vi "Trav_single_profile.vi"(3 "Simulate/Run":T1, 5 "Traverse line":T2 {"Carrier_2 Q (l/min)" format="%#.2f"; "Row Duration (mins)" format="%#.1f"; "Row No" min=0; "Trace Gas Concentration (%)" min=0.0 format="%#_4f"; "Carrier_1 Q (l/min)" format="%#.2f"; "Tunnel Speed" format="%#.2f"; "Start X" format="%#.2f"; "Start Y" format="%#.2f"; "Start Z" format="%#.2f"; "End X" format="%#.2f"; "End Y" format="%#.2f"; "End Z" format="%#.2f"; "Averaging time (min)" min=0.0 format="%#.2f"}) -> (0 "Error Messages":string, 1 "Status":T5, 2 "Traverse line Out":T2 {"Carrier_2 Q (l/min)" format="%#.2f"; "Row Duration (mins)" format="%#.1f"; "Row No" min=0; "Trace Gas Concentration (%)" min=0.0 format="%#_4f"; "Carrier_1 Q (l/min)" format="%#.2f"; "Tunnel Speed" format="%#.2f"; "Start X" format="%#.2f"; "Start Y" format="%#.2f"; "Start Z" format="%#.2f"; "End X" format="%#.2f"; "End Y" format="%#.2f"; "End Z" format="%#.2f"; "Averaging time (min)" min=0.0 format="%#.2f"})   [LabVIEW 2015]
uses:
  Gen Trav/Multi_Run_Status.ctl
  Gen Trav/Traverse_cluster.ctl
  Gen Trav/Spacing.ctl
  Controls/Multi_run_mode.ctl
  Controls/User_Specific_mode.ctl
  Controls/Overhead.ctl
  Controls/Setup.ctl
  Controls/Save_Data.ctl
  Camera Server/Camera enum/Camera resolution.ctl
  ADAM Client/Sub VIs/ADAM Controls/Traverse_Level_State.ctl
  Globals/Extra_Commands_Global.vi
  Globals/Trav_pos_global.vi
  Globals/Meas_global.vi
panel:
  out "Pause message":string
  in  "Pause":bool
  out "Current position":sgl[](array[numeric]) format="%.2f"
  in  "Stop":bool
  in  "Array of Positions":sgl[][](array[numeric]) format="%.2f"
  out "Abcissa copy":string="Y (mm)"
  out "Abcissa":string="Y (mm)"
  in  "ChannelsToPlot":i32[](listbox)=[1]
  out "Started Profile at:":string="16/9/98 12:33"
  out "Currently on point":i32=9
  out "Means":cluster{sgl[], sgl[]}[](graph)
  out "Turbulence%":cluster{sgl[], sgl[]}[](graph)
  # "X           Y            Z"
  # "Start"
  # "End"
  # "X           Y            Z"
  # "Start"
  # "End"
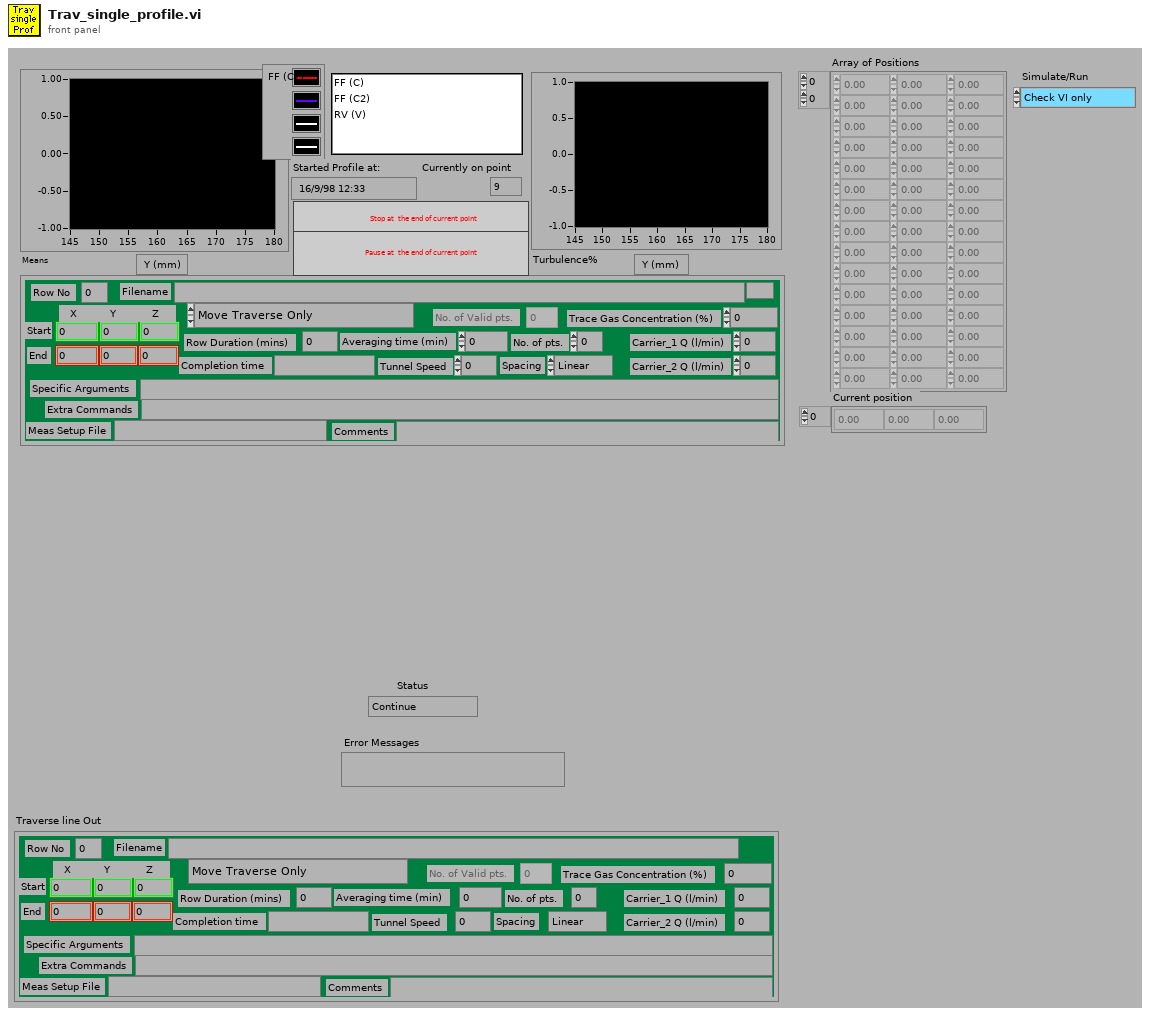
[diagram p1: front panel]
types:
  T1 = typedef "User_Specific_mode.ctl" = enum16{"Check VI only", "Run VI"}
  T2 = typedef "Traverse_cluster.ctl" = cluster{"Start X":sgl, "Start Y":sgl, "Start Z":sgl, "End X":sgl, "End Y":sgl, "End Z":sgl, "No. of pts.":i32, "Spacing":T3, "Filename":path, "Tunnel Speed":dbl, "Averaging time (min)":dbl, "Extra Commands":string, "Carrier_1 Q (l/min)":dbl, "Carrier_2 Q (l/min)":dbl, "Trace Gas Concentration (%)":dbl, "Specific Arguments":string, "Comments":string, "Row No":i32, "Row Type Selector":T4, "Completion time":string, "Row Duration (mins)":dbl, "No. of Valid pts.":i32, "Meas Setup File":string}
  T3 = typedef "Spacing.ctl" = enum16{"Linear", "Log", "Gauss", "Specified", "N/A"}
  T4 = typedef "Multi_run_mode.ctl" = enum16{"Move Traverse Only", "Set Tunnel Speed Only", "Set Source Only", "Set Measurement Conditions", "Single Measurement", "Vertical Profile", "Lateral Profile", "Longitudinal Profile", "Explore Volume", "Multi-Axis Profile", "Auto Calibrate", "Meas Fast FID Bkgnd", "Check Beam Power", "Scanning Valve Measurement", "Run VI Named:", "Set ADAM Ch", "Wait (minutes)", "Send Message", "Synchronize With:", "Fall Back to this Row", "Turn Off Row Repeating", "Blank Row", "Traverse 3D Volume"}
  T5 = typedef "Multi_Run_Status.ctl" = enum16{"Continue", "Jump to Next Point", "Jump to Next Row", "Jump To Fall Back", "Terminate Run"}
  T6 = typedef "Overhead.ctl" = enum16{"Update total times", "Read Current Overhead", "Re Scale totals to 3 hrs", "Initialise totals to 3hr"}
  T7 = typedef "Save_Data.ctl" = enum16{"Save No Data", "Save Data"}
  T8 = typedef "Setup.ctl" = enum16{"Run Program", "Show Setup", "Save Current Setup", "Setup Front Panel"}
  T9 = typedef "Traverse_Level_State.ctl" = enum16{"Running", "Complete"}
  T10 = typedef "Status_Cluster.ctl" = cluster{"Status":T5, "Error Type":string, "Error Description":string}
  T11 = typedef "Camera resolution.ctl" = u8
  T12 = typedef "Analysis_info_cluster.ctl" = cluster{"Colour":u32, "Inst type":T13, "Inst name":string, "Symbol":string, "Code name":string, "Extra Info":string, "Inst Array":T14, "Extra Titles":string[], "Extra Values":string[], "U":dbl, "u^2":dbl, "u^3":dbl, "u^4":dbl, "Skew_u":dbl, "Kurt_u":dbl, "Sd Error in Mean":dbl, "% u'/U":dbl, "X":dbl, "Y":dbl, "Z":dbl, "Timescale integral to 25%":dbl, "Sd Error in Variance":dbl, "Calib File":path, "Calib Constants":dbl[], "Output Position":bool, "Full Stats":bool, "Av Sampling Rate":dbl, "Av No of Samples":dbl, "Total Meas Time (s)":dbl, "ADAM Ch Name":string, "Max value":dbl, "Min value":dbl}
  T13 = typedef "Inst_type.ctl" = enum16{"Propeller anemometer", "Raw voltage", "Pressure Transducer", "Pitot-static tube", "Preston tube", "Hot wire", "Cross wire 1", "Cross wire 2", "Generic Linear", "Generic Polynomial", "Generic BackPoly", "Fast FID", "Thermocouple", "Cold wire", "Pulsed Wire", "LDA Vel", "LDA Tran time", "LDA Arr time", "Microphone"}
  T14 = typedef "Instrument_Array.ctl" = enum16{"PWA", "LDA", "Analogue"}
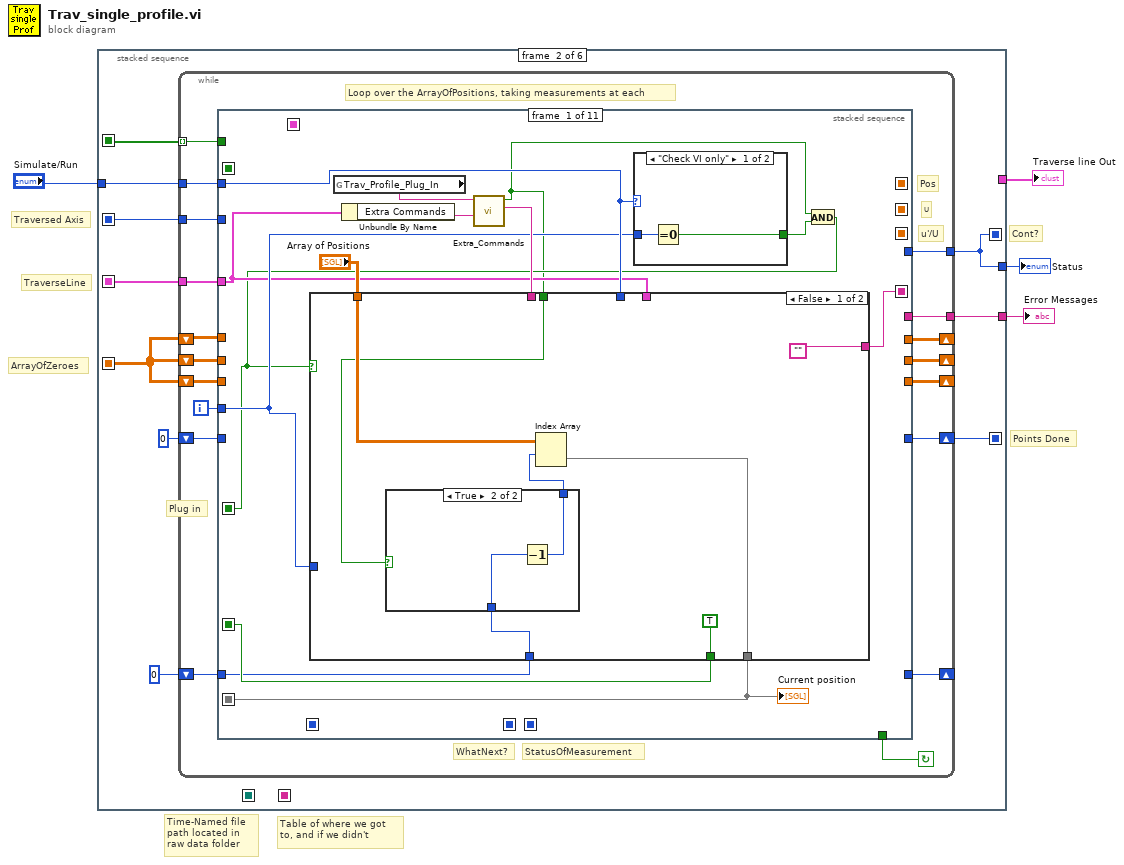
[diagram p0: block diagram]
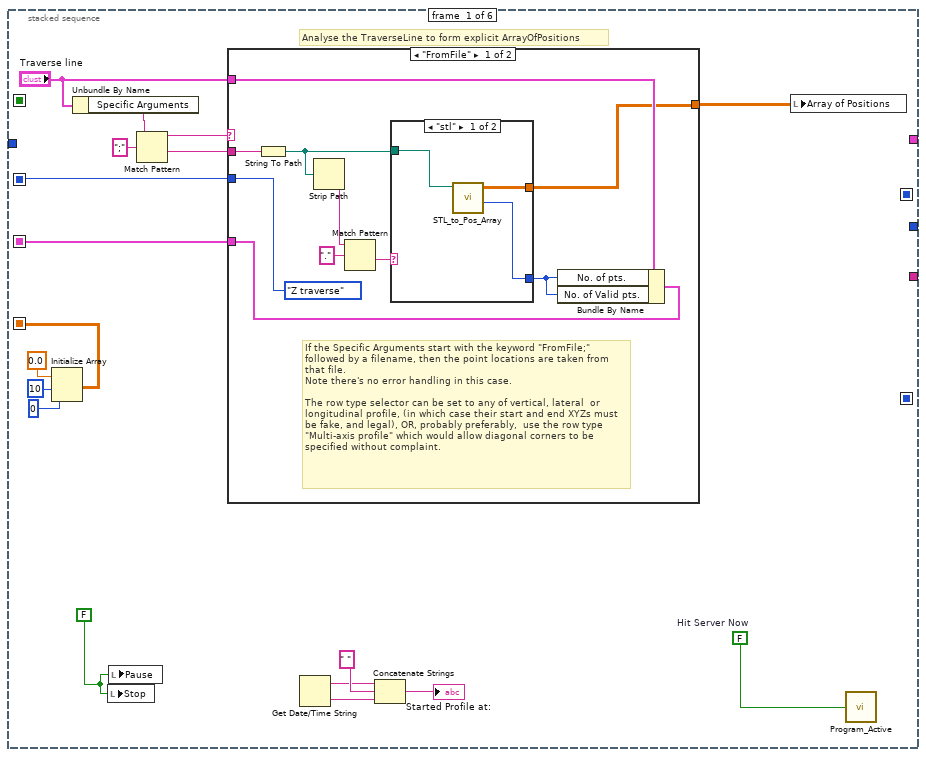
[diagram p2: hidden frame]
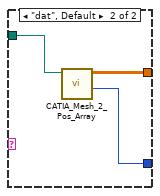
[diagram p3: hidden frame]
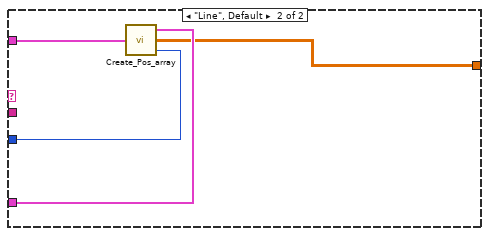
[diagram p4: hidden frame]
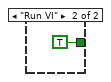
[diagram p5: hidden frame]
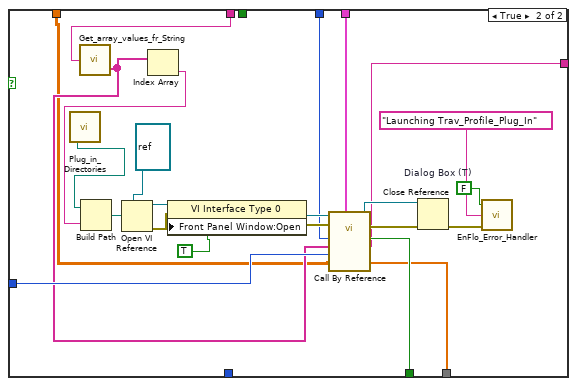
[diagram p7: hidden frame]
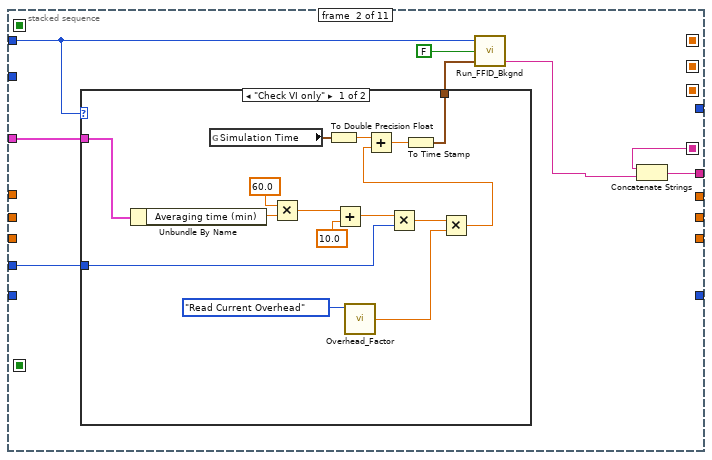
[diagram p8: hidden frame]
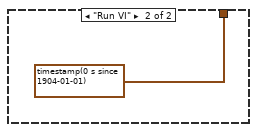
[diagram p9: hidden frame]
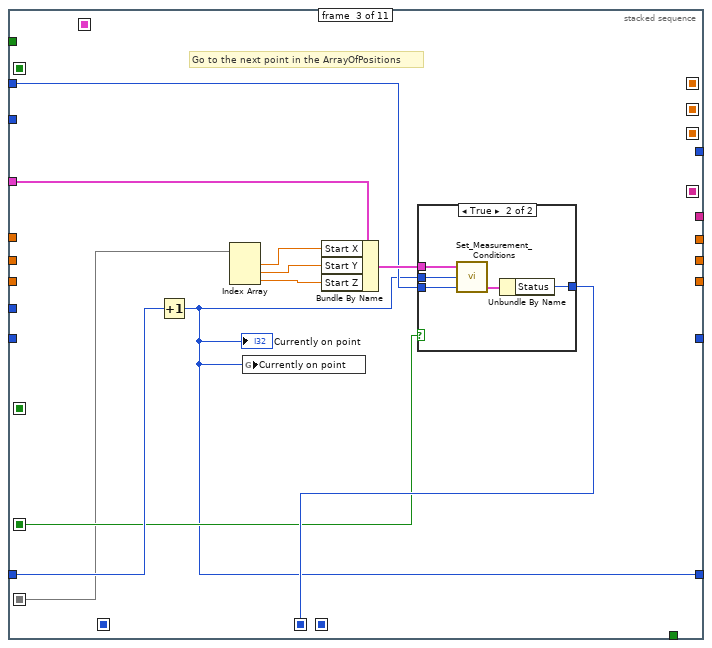
[diagram p10: hidden frame]
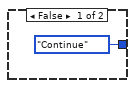
[diagram p11: hidden frame]
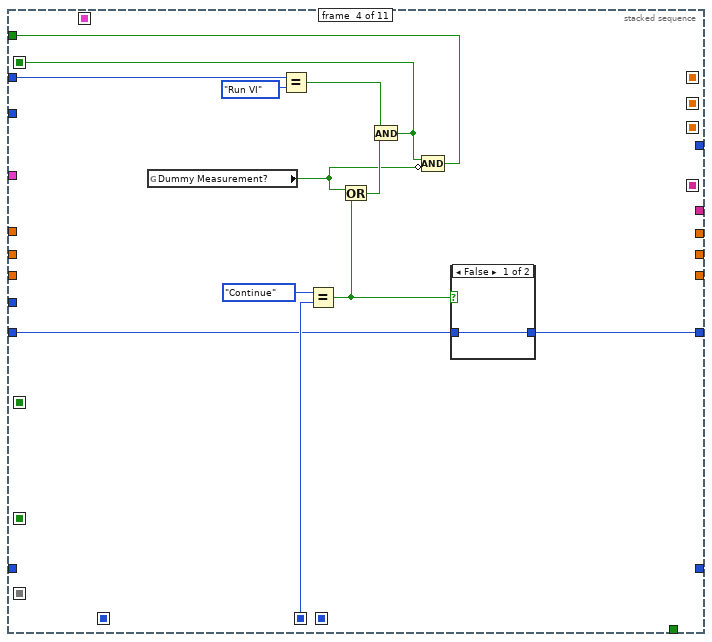
[diagram p12: hidden frame]
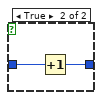
[diagram p13: hidden frame]
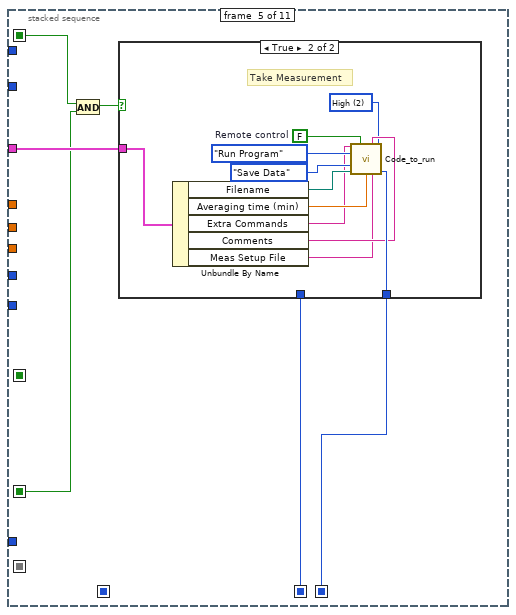
[diagram p14: hidden frame]
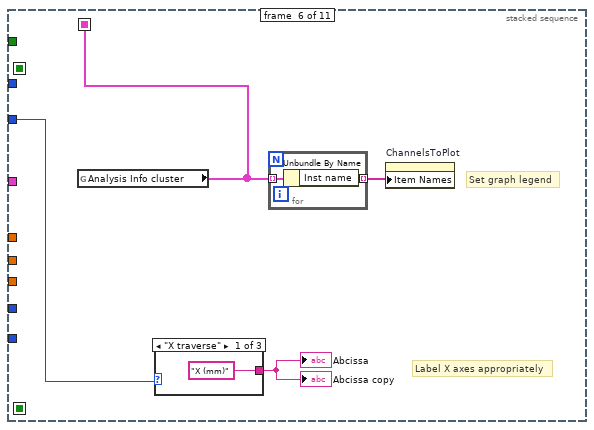
[diagram p16: hidden frame]
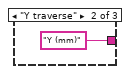
[diagram p17: hidden frame]
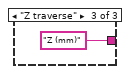
[diagram p18: hidden frame]
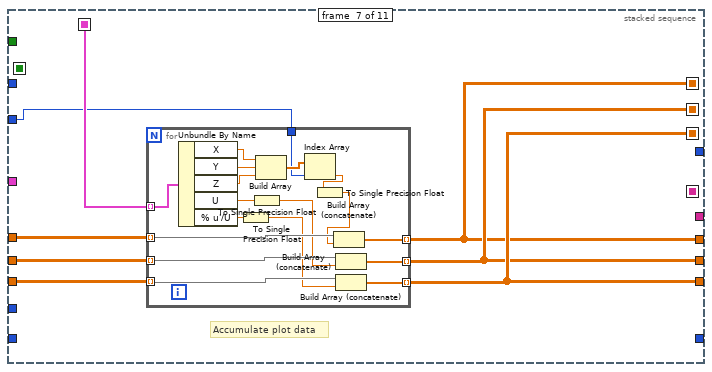
[diagram p19: hidden frame]
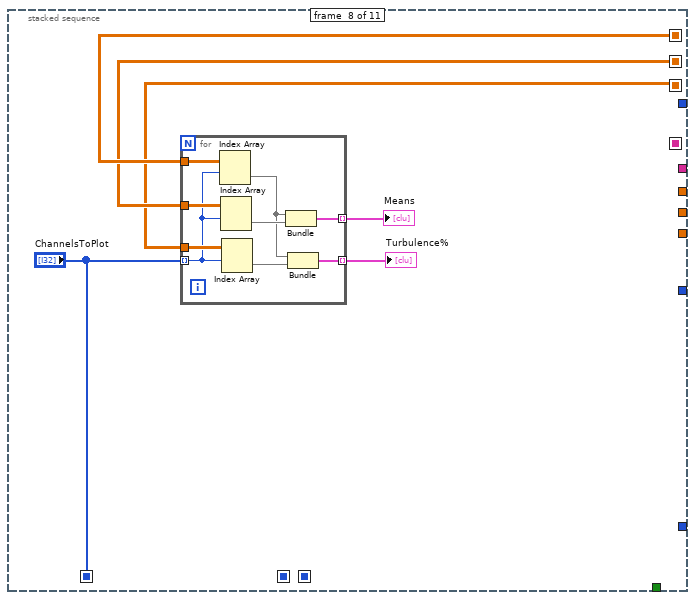
[diagram p20: hidden frame]
diagram:
  # "Table of where we got to, and if we didn't"
  # "Time-Named file path located in raw data folder"
  # "ArrayOfZeroes"
  # "TraverseLine"
  # "Traversed Axis"
  # "Points Done"
  # "Cont?"
  n1 = stacked-sequence {
    seq-local: [w15 _ _ _ _ _] -> [_ w51 _ _ _ _]
    seq-local: [w14 _ _ _ _ _] -> [_ w52 _ _ _ _]
    seq-local: [_ _ w335 _ _ _] -> [_ _ _ _ w359 _]
    seq-local: [_ _ _ w342 _ _] -> [_ _ _ _ w358 _]
    seq-local: [_ w50 _ _ _ _] -> [_ _ _ _ _ _]
    seq-local: [_ w48 _ _ _ _] -> [_ _ _ w339 w357 _]
    seq-local: [_ w46 _ _ _ _] -> [_ _ _ _ _ w364]
    seq-local: [w11 _ _ _ _ _] -> [_ w45 _ _ _ w366]
    tunnel: [_ w50 _ _ _ _] -> w2
    tunnel: [_ _ _ _ _ w376] -> w4
    tunnel: "Simulate/Run" -> [_ w49 _ _ _ w375]
    tunnel: [_ w44 _ _ _ _] -> w1
    frame #0 {
      w12 = FALSE ("stop")
      w13 = FALSE  # Hit Server Now
      # "Analyse the TraverseLine to form explicit ArrayOfPositions"
      n2 = Initialize Array(sgl 0.0, 10, 0) -> (w15:sgl[][])
      n3 = Unbundle By Name("Traverse line") -> ("Specific Arguments"=w8:string)
      n4 = local write "Stop"(w12) -> ()
      n5 = local write "Pause"(w12) -> ()
      n6 = Match Pattern(string=w8, regular expression=";") -> (before substring=w6:string, after substring=w5:string)  [unwired: 1 in, 2 out]
      n7 = case shown="\"FromFile\"" w6 {
        tunnel: [enum16{"X traverse", "Y traverse", "Z traverse"}."Z traverse" ("Axis Traversed") w42] -> w14
        tunnel: "Traverse line" -> [w26 w41]
        tunnel: [w25 w40] -> w11
        tunnel: [w23 w39] -> w10
        tunnel: w5 -> [w27 _]
        frame "FromFile" {
          # "If the Specific Arguments start with the keyword \"FromFile;\" followed by a filename, then the point locations are taken from that file.\nNote there's no error handling in this case.\n\nThe row type selector can be set to any of vertical, lateral  or longitudinal profile, (in which case their start and end XYZs must be fake, and legal), OR, probably preferably,  use the row type \"Multi-axis profile\" which would allow diagonal corners to be specified without complaint."
          n8 = String To Path(string=w27) -> (path=w29:path)
          n9 = Strip Path(path=w29) -> (name=w31:string)  [unwired: 1 out]
          n10 = Match Pattern(string=w31, regular expression=".") -> (after substring=w32:string)  [unwired: 1 in, 3 out]
          n11 = case shown="\"stl\"" w32 {
            tunnel: [w34 w38] -> w23
            tunnel: [w33 w37] -> w28
            tunnel: w29 -> [w35 w36]
            frame "stl" {
              n12 = call "STL_to_Pos_Array.vi"("STL file"=w35) -> ("Number of Points"=w33:i32, "Array of Positions"=w34:dbl[][])  [unwired: 9 in]
            }
            frame "dat", Default {
              n13 = call "CATIA_Mesh_2_Pos_Array.vi"("Catia Mesh File"=w36) -> ("Number of Points"=w37:i32, "Array of Positions"=w38:dbl[][])  [unwired: 9 in]
            }
          }
          n14 = Bundle By Name(cluster=w26, "No. of pts."=w28, "No. of Valid pts."=w28) -> (w25:T2)
        }
        frame "Line", Default {
          n15 = call "Create_Pos_array.vi"("Traverse line"=w41) -> ("Traverse line Out"=w40:T2, "Array of Positions"=w39:dbl[][], "Axis Traversed"=w42:enum16{"X traverse", "Y traverse", "Z traverse"})  [unwired: 5 in, 1 out]
        }
      }
      n16 = Get Date/Time String() -> (date string=w21:string, time string=w20:string)  [unwired: 3 out]
      n17 = Concatenate Strings(w21, " ", w20) -> (→"Started Profile at:":string)
      n18 = local write "Array of Positions"(w10) -> ()
      n19 = call "Program_Active.vi"("Hit Server Now"=w13) -> ()
    }
    frame #1 {
      # "Plug in"
      n20 = while {
        shift-left: 0 -> [w57]
        shift-right: [w56] -> w46
        tunnel: [w58] -> w48 mode=indexing
        tunnel: w45 -> [w59]
        tunnel: w49 -> [w60]
        tunnel: [w61] -> w50
        shift-left: w51 -> [w64]
        shift-right: [w63] -> _
        tunnel: w52 -> [w65]
        shift-left: w51 -> [w67]
        shift-right: [w66] -> _
        shift-left: w51 -> [w69]
        shift-right: [w68] -> _
        tunnel: [w55] -> w44
        shift-right: [w53] -> _
        shift-left: 0 -> [w54]
        i -> [w70]
        stop <- w62 continue-if-true
        # "StatusOfMeasurement"
        # "WhatNext?"
        # "Loop over the ArrayOfPositions, taking measurements at each"
        # "Pos"
        # "U"
        # "u'/U"
        n21 = stacked-sequence {
          seq-local: [_ _ _ _ _ w195 _ _ _ _ _] -> [_ _ _ _ _ _ w209 _ w245 _ _]
          seq-local: [_ _ _ _ _ _ w205 _ _ _ _] -> [_ _ _ _ _ _ _ w235 _ _ _]
          seq-local: [_ _ _ _ _ _ w207 _ _ _ _] -> [_ _ _ _ _ _ _ w234 _ _ _]
          seq-local: [_ _ _ _ _ _ w208 _ _ _ _] -> [_ _ _ _ _ _ _ w233 _ _ _]
          seq-local: [_ _ _ _ _ _ _ "ChannelsToPlot" _ _ _] -> [_ _ _ _ _ _ _ _ w251 _ _]
          seq-local: [_ _ _ _ w182 _ _ _ _ _ _] -> [_ _ _ _ _ _ _ _ _ _ w311]
          seq-local: [_ _ w151 _ _ _ _ _ _ _ _] -> [_ _ _ w171 w181 _ _ _ _ _ _]
          seq-local: [_ _ _ w163 _ _ _ _ _ _ _] -> [_ _ _ _ w179 _ _ _ _ _ _]
          seq-local: [w81 _ _ _ _ _ _ _ _ _ _] -> [_ _ w147 _ w178 _ _ _ _ _ w307]
          seq-local: [w80 _ _ _ _ _ _ _ _ _ _] -> [_ w125 _ _ _ _ _ _ _ _ _]
          seq-local: [w75 _ _ _ _ _ _ _ _ _ _] -> [_ _ w146 _ _ _ _ _ _ _ _]
          seq-local: [w72 _ _ _ _ _ _ _ _ _ _] -> [_ _ _ _ _ _ _ _ _ _ w304]
          tunnel: w70 -> [w78 w126 _ _ _ _ _ _ _ _ _]
          tunnel: w69 -> [_ _ _ _ _ _ w211 _ _ _ _]
          tunnel: [_ _ _ _ _ _ w207 _ _ _ _] -> w68
          tunnel: w67 -> [_ _ _ _ _ _ w210 _ _ _ _]
          tunnel: [_ _ _ _ _ _ w208 _ _ _ _] -> w66
          tunnel: w65 -> [_ _ _ _ _ w197 w204 _ _ _ _]
          tunnel: w64 -> [_ _ _ _ _ _ w206 _ _ _ _]
          tunnel: [_ _ _ _ _ _ w205 _ _ _ _] -> w63
          tunnel: [_ _ _ _ _ _ _ _ _ _ w306] -> w62
          tunnel: w59 -> [w74 w127 w154 _ w180 _ _ _ _ _ _]
          tunnel: [_ _ _ _ _ _ _ _ _ _ w305] -> w61
          tunnel: w60 -> [w79 w128 w152 w173 _ _ _ _ _ _ _]
          tunnel: [_ _ _ w164 _ _ _ _ _ _ _] -> w58
          tunnel: w57 -> [_ _ _ w168 _ _ _ _ _ _ _]
          tunnel: [_ _ _ w167 _ _ _ _ _ _ _] -> w56
          tunnel: [_ w123 _ _ _ _ _ _ _ _ _] -> w55
          tunnel: w54 -> [w73 _ w148 _ _ _ _ _ _ _ w303]
          tunnel: [_ _ w145 _ _ _ _ _ _ _ _] -> w53
          frame #0 {
            n22 = global read "Extra_Commands_Global.vi" "Trav_Profile_Plug_In"() -> (w84:string)
            n23 = Unbundle By Name(w74) -> ("Extra Commands"=w83:string)
            n24 = call "Extra_Commands.vi"("String to Search"=w83, "Command"=w84) -> ("String Value"=w82:string, "Command Found"=w71:bool)  [unwired: 1 in, 3 out]
            n25 = case shown="\"Check VI only\"" w79 {
              tunnel: w78 -> [w86 _]
              tunnel: [w85 TRUE] -> w77
              frame "Check VI only" {
                n26 = Equal To 0?(x=w86) -> (x = 0?=w85:bool)
              }
              frame "Run VI" {
              }
            }
            n27 = And(x=w71, y=w77) -> (x .and. y?=w72:bool)
            n28 = case shown="False" w72 {
              tunnel: w82 -> [_ w119]
              tunnel: w78 -> [_ w105]
              tunnel: [TRUE ("Stop") w104] -> w81
              tunnel: w79 -> [_ w103]
              tunnel: ["" w101] -> w80
              tunnel: w73 -> [w89 _]
              tunnel: "Array of Positions" -> [w92 w100]
              tunnel: [w91 w99] -> w75
              tunnel: w74 -> [_ w98]
              tunnel: w71 -> [w90 _]
              frame False {
                n29 = case shown="True" w90 {
                  tunnel: w89 -> [w95 w97]
                  tunnel: [w95 w96] -> w88
                  frame False {
                  }
                  frame True {
                    n30 = Decrement(x=w97) -> (x-1=w96:i32)
                  }
                }
                n31 = Index Array(array=w92, index (row)=w88) -> (element=w91:sgl[])  [unwired: 1 in]
              }
              frame True {
                w115 = FALSE  # Dialog Box (T)
                n32 = call "Plug_in_Directories.vi"() -> ("Trav_Profile_Plug_Ins"=w120:path)  [unwired: 2 in, 4 out]
                n33 = call "Get_array_values_fr_String.vi"("String Value"=w119) -> ("String array"=w102:string[])  [unwired: 1 out]
                n34 = Index Array(array=w102) -> (element=w118:string)  [unwired: 1 in]
                n35 = Build Path(base path=w120, name or relative path=w118) -> (appended path=w110:path)
                n36 = Open VI Reference(type specifier VI Refnum (for type only)=refnum<vi> refnum ("Plug in"), vi path=w110) -> (vi reference=w113:refnum<vi>, error out=w112:errorcluster)  [unwired: 2 in, 2 out]
                n37 = property class="VI Interface Type 0"(reference=w113, error in=w112, "Front Panel Window:Open"=TRUE ("Wait until done")) -> (reference out=w109:refnum<vi>, error out=w108:errorcluster)
                n38 = call-by-ref "?"(reference=w109, error in=w108, "Traverse line"=w98, "Array of Positions"=w100, "Loop i"=w105, "Arguments"=w102, "Simulate/Run"=w103) -> (reference out=w107:refnum<vi>, error out=w106:errorcluster, "Next Position"=w99:sgl[], "Error String"=w101:string, "Continue"=w104:bool)  [unwired: 1 in]
                n39 = Close Reference(reference=w107, error in (no error)=w106) -> (error out=w116:errorcluster)
                n40 = call "EnFlo_Error_Handler.vi"("error in (no error)"=w116, "Error Type"="Launching Trav_Profile_Plug_In", "Dialog Box (T)"=w115) -> ()  [unwired: 3 out]
              }
            }
            "Current position" <- w75
          }
          frame #1 {
            n41 = case shown="\"Check VI only\"" w128 {
              tunnel: w127 -> [w143 _]
              tunnel: w126 -> [w129 _]
              tunnel: [w132 timestamp(0 s since 1904-01-01)] -> w122
              frame "Check VI only" {
                n42 = Unbundle By Name(w143) -> ("Averaging time (min)"=w140:dbl)
                n43 = global read "Trav_pos_global.vi" "Simulation Time"() -> (w134:timestamp)
                n44 = Multiply(x=60.0, y=w140) -> (x*y=w139:dbl)
                n45 = To Double Precision Float(number=w134) -> (double precision float=w135:dbl)
                n46 = Add(x=w139, y=10.0 ("Scalable Time (Sec)")) -> (x+y=w138:dbl)
                n47 = call "Overhead_Factor.vi"("Mode"=Overhead."Read Current Overhead") -> ("Current Overhead Factor"=w130:dbl)  [unwired: 3 in]
                n48 = Multiply(x=w138, y=w129) -> (x*y=w131:dbl)
                n49 = Multiply(x=w131, y=w130) -> (x*y=w136:dbl)
                n50 = Add(x=w135, y=w136) -> (x+y=w133:dbl)
                n51 = To Time Stamp(1:w133) -> (0:w132:timestamp)
              }
              frame "Run VI" {
              }
            }
            n52 = call "Run_FFID_Bkgnd.vi"("Simulated Time"=w122, "Run Now?"=FALSE, "Simulate/Run"=w128) -> ("Error Messages"=w124:string)  [unwired: 2 out]
            n53 = Concatenate Strings(w125, w124) -> (w123:string)
          }
          frame #2 {
            # "Go to the next point in the ArrayOfPositions"
            n54 = Increment(x=w148) -> (x+1=w145:i32)
            "Currently on point" <- w145
            n55 = Index Array(array=w146) -> (element #1=w155:sgl, element #2=w150:sgl, element #3=w149:sgl)  [unwired: 3 in]
            n56 = global write "Trav_pos_global.vi" "Currently on point"(w145) -> ()
            n57 = Bundle By Name(cluster=w154, "Start X"=w155, "Start Y"=w150, "Start Z"=w149) -> (w153:T2)
            n58 = case shown="True" w147 {
              tunnel: w153 -> [_ w161]
              tunnel: w152 -> [_ w160]
              tunnel: [Multi_Run_Status."Continue" ("Status") w158] -> w151
              tunnel: w145 -> [_ w157]
              frame False {
              }
              frame True {
                n59 = call "Set_Measurement_Conditions.vi"("Simulate/Run"=w160, "Currently on Point"=w157, "Traverse line"=w161) -> ("Status Cluster"=w159:T10)  [unwired: 2 out]
                n60 = Unbundle By Name(w159) -> ("Status"=w158:T5)
              }
            }
          }
          frame #3 {
            n61 = global read "Trav_pos_global.vi" "Dummy Measurement?"() -> (w162:bool)
            n62 = Equal?(x=w173, y=User_Specific_mode."Run VI" ("Simulate/Run")) -> (x = y?=w169:bool)
            n63 = Equal?(x=Multi_Run_Status."Continue" ("Status"), y=w171) -> (x = y?=w166:bool)
            n64 = Or(x=w162, y=w166) -> (x .or. y?=w165:bool)
            n65 = And(x=w169, y=w165) -> (x .and. y?=w163:bool)
            n66 = Compound Arithmetic op=AND(w163, invert w162) -> (w164:bool)
            n67 = case shown="False" w166 {
              tunnel: w168 -> [w174 w176]
              tunnel: [w174 w175] -> w167
              frame False {
              }
              frame True {
                n68 = Increment(x=w176) -> (x+1=w175:i32)
              }
            }
          }
          frame #4 {
            n69 = And(x=w179, y=w178) -> (x .and. y?=w177:bool)
            n70 = case shown="True" w177 {
              tunnel: [w183 w194] -> w182
              tunnel: w181 -> [w183 _]
              tunnel: w180 -> [_ w188]
              frame False {
                # "Dummy measurement, or some other reason not to actually measure"
              }
              frame True {
                w185 = T11 2 items=["Low", "Med.", "High", "Max."] ("Camera Resolution")
                w193 = FALSE  # Remote control
                # "Take Measurement"
                n71 = Unbundle By Name(w188) -> ("Filename"=w191:path, "Averaging time (min)"=w192:dbl, "Extra Commands"=w187:string, "Comments"=w186:string, "Meas Setup File"=w184:string)
                n72 = call "Code_to_run.vi"("Extra command String"=w187, "Current Row Comments"=w186, "Camera Resolution"=w185, "setup"=Setup."Run Program", "Remote control"=w193, "File"=Save_Data."Save Data", "Results Filename"=w191, "Averaging time (min)"=w192, "Setup filename"=w184) -> ("Status"=w194:T5)  [unwired: 3 in, 3 out]
              }
            }
          }
          frame #5 {
            # "Label X axes appropriately"
            # "Set graph legend"
            n73 = global read "Meas_global.vi" "Analysis Info cluster"() -> (w195:T12[])
            n74 = case shown="\"X traverse\"" w197 {
              tunnel: ["X (mm)" "Y (mm)" "Z (mm)"] -> w196
              frame "X traverse" {
              }
              frame "Y traverse" {
              }
              frame "Z traverse" {
              }
            }
            "Abcissa" <- w196
            "Abcissa copy" <- w196
            n75 = for {
              tunnel: w195 -> [w203] mode=indexing
              tunnel: [w202] -> w198 mode=indexing
              n76 = Unbundle By Name(w203) -> ("Inst name"=w202:string)
            }
            n77 = property on="ChannelsToPlot" class="LstBox (strict)"("Item Names"=w198) -> ()  [unwired: 2 in, 2 out]
          }
          frame #6 {
            # "Accumulate plot data"
            n78 = for {
              tunnel: w211 -> [w229] mode=indexing
              tunnel: [w227] -> w207 mode=indexing
              tunnel: w210 -> [w226] mode=indexing
              tunnel: [w224] -> w208 mode=indexing
              tunnel: w209 -> [w223] mode=indexing
              tunnel: w206 -> [w222] mode=indexing
              tunnel: [w221] -> w205 mode=indexing
              tunnel: w204 -> [w216]
              n79 = Unbundle By Name(w223) -> ("X"=w220:dbl, "Y"=w219:dbl, "Z"=w218:dbl, "U"=w228:dbl, "% u'/U"=w225:dbl)
              n80 = To Single Precision Float(number=w225) -> (single precision float=w214:sgl)
              n81 = To Single Precision Float(number=w228) -> (single precision float=w215:sgl)
              n82 = Build Array(w220, w219, w218) -> (w217:dbl[])
              n83 = Index Array(array=w217, index=w216) -> (element=w213:dbl)
              n84 = To Single Precision Float(number=w213) -> (single precision float=w212:sgl)
              n85 = Build Array (concatenate)(w222, w212) -> (w221:sgl[])
              n86 = Build Array (concatenate)(w229, w215) -> (w227:sgl[])
              n87 = Build Array (concatenate)(w226, w214) -> (w224:sgl[])
            }
          }
          frame #7 {
            n88 = for {
              tunnel: "ChannelsToPlot" -> [w236] mode=indexing
              tunnel: w235 -> [w244]
              tunnel: w234 -> [w243]
              tunnel: w233 -> [w242]
              tunnel: [w238] -> w232 mode=indexing
              tunnel: [w237] -> w231 mode=indexing
              n89 = Index Array(array=w244, index (row)=w236) -> (element=w240:sgl[])  [unwired: 1 in]
              n90 = Index Array(array=w243, index (row)=w236) -> (element=w241:sgl[])  [unwired: 1 in]
              n91 = Index Array(array=w242, index (row)=w236) -> (element=w239:sgl[])  [unwired: 1 in]
              n92 = Bundle(w240, w241) -> (w237:cluster{sgl[], sgl[]})  [unwired: 1 out]
              n93 = Bundle(w240, w239) -> (w238:cluster{sgl[], sgl[]})  [unwired: 1 out]
            }
            "Means" <- w231
            "Turbulence%" <- w232
          }
          frame #8 {
            # "add some empty plot names"
            n94 = for {
              tunnel: w251 -> [w255] mode=indexing
              tunnel: w245 -> [w253]
              tunnel: [w252] -> w248 mode=indexing
              n95 = Index Array(array=w253, index=w255) -> (element=w254:T12)
              n96 = Unbundle By Name(w254) -> ("Inst name"=w252:string)
            }
            n97 = Initialize Array("", 5) -> (w247:string[])
            n98 = Build Array (concatenate)(w248, w247) -> (w246:string[])
            n99 = for {
              tunnel: w246 -> [w256] mode=indexing
              i -> [w258]
              n100 = To Unsigned Long Integer(number=w258) -> (unsigned 32bit integer=w257:u32)
              n101 = property on="Means" class="XYGraph (strict)"("Active Plot"=w257, "Plot.Plot Name"=w256) -> ()  [unwired: 2 in, 2 out]
              n102 = property on="u'/U" class="XYGraph (strict)"("Active Plot"=w257, "Plot.Plot Name"=w256) -> ()  [unwired: 2 in, 2 out]
            }
          }
          frame #9 {
            w259 = -1
            # "Check in with server, and pause if requested"
            n103 = while {
              shift-left: w259 -> [w260]
              shift-right: [w261] -> _
              shift-left: w259 -> [w264]
              shift-right: [w265] -> _
              stop <- w262 continue-if-true
              n104 = Increment(x=w264) -> (x+1=w263:i32)
              n105 = case shown="4" w264 {
                tunnel: [w270 w273 w277 w287 w290 w294 0] -> w265
                tunnel: w263 -> [w270 w273 w279 w287 w290 w294 _]
                tunnel: [TRUE ("Pause") "Pause" TRUE ("Pause") TRUE ("Pause") TRUE ("Pause") TRUE ("Pause") TRUE ("Pause")] -> w262
                tunnel: [w269 w272 w275 w284 w288 w292 w297] -> w261
                tunnel: w260 -> [w269 w272 w275 w284 w288 w292 w298]
                frame -1 {
                  # "Report to server"
                  n106 = call "Program_Active_Client.vi"("Mode"=enum16{"Program Active", "Traverse Level State"}."Program Active", "Time till next contact (Sec)"=12000.0, "Traverse level State"=Traverse_Level_State."Running") -> ()  [unwired: 3 out]
                }
                frame 0, Default {
                  # "If user wants to pause..."
                }
                frame 1 {
                  n107 = Quotient & Remainder(x=w275, y=15) -> (x-y*floor(x/y)=w281:i32)  [unwired: 1 out]
                  n108 = global write "Trav_pos_global.vi" "Paused During Row?"(TRUE ("Paused During Row?")) -> ()
                  n109 = Equal To 0?(x=w281) -> (x = 0?=w280:bool)
                  n110 = Increment(x=w279) -> (x+1=w278:i32)
                  n111 = Select(t=w279, s=w280, f=w278) -> (s? t:f=w277:i32)
                }
                frame 2 {
                  # "Bring to front occasionally to remind user we're paused"
                  n112 = Current VI's Path() -> (path=w285:path)
                  n113 = call "Bring_to_front.vi"("path"=w285) -> ()
                }
                frame 3 {
                  # "Write to big indcator, and then flash on and off"
                  "Pause message" <- "Multi Run Program Paused!!!!" ("Pause message")
                }
                frame 4 {
                  n114 = property on="Pause message" class="Str"("Visible"=TRUE) -> ()  [unwired: 2 in, 2 out]
                  n115 = Wait Until Next ms Multiple(millisecond multiple=u32 1500) -> ()  [unwired: 1 out]
                }
                frame 5 {
                  n116 = Increment(x=w298) -> (x+1=w297:i32)
                  n117 = property on="Pause message" class="Str"("Visible"=FALSE) -> ()  [unwired: 2 in, 2 out]
                  n118 = Wait Until Next ms Multiple(millisecond multiple=u32 1500) -> ()  [unwired: 1 out]
                }
              }
            }
          }
          frame #10 {
            n119 = case shown="False" w304 {
              tunnel: [w315 TRUE] -> w309
              tunnel: w303 -> [w314 _]
              frame False {
                n120 = local read "Array of Positions"() -> (w316:sgl[][])
                n121 = Array Size(array=w316) -> (size(s)=w319:i32[])
                n122 = Index Array(array=w319, index=0 ("Index")) -> (element=w317:i32)
                n123 = Increment(x=w314) -> (x+1=w313:i32)
                n124 = Less?(x=w313, y=w317) -> (x < y?=w315:bool)
              }
              frame True {
              }
            }
            n125 = case shown="\"Jump to Next Point\"" w311 {
              tunnel: [TRUE TRUE FALSE] -> w308
              frame "Continue" {
              }
              frame "Jump to Next Point" {
              }
              frame "Jump to Next Row", Default {
              }
            }
            n126 = Compound Arithmetic op=AND(invert "Stop", w309, w308, w307) -> (w306:bool)
            n127 = Select(t=Multi_Run_Status."Terminate Run" ("Status"), s="Stop", f=w311) -> (s? t:f=w305:T5)
          }
        }
      }
    }
    frame #2 {
      n128 = global read "Meas_global.vi" "Start Time of experiment"() -> (w325:dbl)
      n129 = global read "Meas_global.vi" "Raw data file"() -> (w337:path)
      n130 = Strip Path(path=w337) -> (stripped path=w336:path)  [unwired: 1 out]
      n131 = call "Sec_to_date_filename.vi"("seconds"=w325) -> ("Day"=w327:string, "Time"=w328:string)  [unwired: 2 out]
      n132 = Format Into String(format string="Cmd_%s_%s.xls", w327, w328) -> (resulting string=w330:string)  [unwired: 2 in, 1 out]
      n133 = call "Fast_string_Replace.vi"("Replace match with:"="-", "Input String"=w330, "regular expression"=":") -> ("Output String"=w333:string)  [unwired: 2 out]
      n134 = call "Fast_string_Replace.vi"("Replace match with:"="", "Input String"=w333, "regular expression"=" ") -> ("Output String"=w324:string)  [unwired: 2 out]
      n135 = Build Path(base path=w336, name or relative path=w324) -> (appended path=w335:path)
    }
    frame #3 {
      w348 = "\t"
      n136 = local read "Array of Positions"() -> (w341:sgl[][])
      n137 = Number To Fractional String(number=w341, precision (6)=i16 2) -> (F-format string=w340:string[][])  [unwired: 2 out]
      n138 = for {
        tunnel: w340 -> [w353] mode=indexing
        tunnel: w339 -> [w352] mode=indexing
        tunnel: [w350] -> w338 mode=indexing
        n139 = case shown="True" w352 {
          tunnel: ["Unobtainable Position" ""] -> w351
          frame False {
          }
          frame True {
          }
        }
        n140 = Build Array (concatenate)(w353, w351) -> (w350:string[])
      }
      n141 = Concatenate Strings("X", w348, "Y", w348, "Z") -> (w343:string)
      n142 = call "2D_array_to_string.vi"("2D data array"=w338, "Column titles  (separated by tabs)"=w343, "Array title"="Requested positions") -> ("Output string"=w342:string)
    }
    frame #4 {
      n143 = Or Array Elements(Boolean array=w357) -> (logical OR=w356:bool)
      n144 = case shown="True" w356 {
        tunnel: w359 -> [_ w362]
        tunnel: w358 -> [_ w360]
        frame False {
        }
        frame True {
          w361 = FALSE  # Lock File
          w363 = TRUE  # append to file? (new file:F)
          # "If we managed to get to even one point, write a file"
          n145 = call "Write_Characters_To_File.vi"("file path (dialog if empty)"=w362, "character string"=w360, "append to file? (new file:F)"=w363, "Lock File"=w361) -> ()  [unwired: 1 in, 4 out]
        }
      }
    }
    frame #5 {
      n146 = local read "Array of Positions"() -> (w368:sgl[][])
      n147 = Array Size(array=w368) -> (size(s)=w370:i32[])
      n148 = Index Array(array=w370, index=0 ("Index")) -> (element=w367:i32)
      n149 = Not Equal?(x=w367, y=w364) -> (x != y?=w373:bool)
      n150 = Equal?(x=User_Specific_mode."Run VI" ("Simulate/Run"), y=w375) -> (x = y?=w372:bool)
      n151 = Bundle By Name(cluster=w366, "No. of Valid pts."=w364) -> (w365:T2)
      n152 = And(x=w372, y=w373) -> (x .and. y?=w371:bool)
      n153 = case shown="True" w371 {
        tunnel: w365 -> [w377 w389]
        tunnel: [w377 w388] -> w376
        tunnel: w364 -> [_ w387]
        frame False {
        }
        frame True {
          w378 = " !!Program added comments"
          n154 = Unbundle By Name(w389) -> ("Comments"=w379:string)
          n155 = Equal To 0?(x=w387) -> (x = 0?=w386:bool)
          n156 = Select(t=" !!(Row Skipped)", s=w386, f=" !!(Row Partially Skipped)") -> (s? t:f=w382:string)
          n157 = Match Pattern(string=w379, regular expression=w378) -> (match substring=w381:string)  [unwired: 4 out]
          n158 = Empty String/Path?(string/path=w381) -> (empty?=w380:bool)
          n159 = case shown="False" w380 {
            tunnel: [w392 w396] -> w383
            tunnel: w382 -> [w391 w395]
            tunnel: w378 -> [_ w394]
            tunnel: w379 -> [w390 w393]
            frame False {
              n160 = Concatenate Strings(w390, w391) -> (w392:string)
            }
            frame True {
              n161 = Concatenate Strings(w393, w394, w395) -> (w396:string)
            }
          }
          n162 = Bundle By Name(cluster=w389, "Comments"=w383) -> (w388:T2)
        }
      }
    }
  }
  "Status" <- w2
  "Traverse line Out" <- w4
  "Error Messages" <- w1
